vi "set led intensity.vi"(0 "WindowHandle in":T1, 2 "Abort Ref":refnum<vi>, 5 "HWND in":u32, 7 "LED":enum16{"5", "6", "10", "13", "24", "28"}(ring), 9 "PIN setpoint":i32=100, 11 "error in":errorcluster) -> (4 "WindowHandle out":T1, 6 "HWND out":u32, 15 "error out":errorcluster)   [LabVIEW 2018]
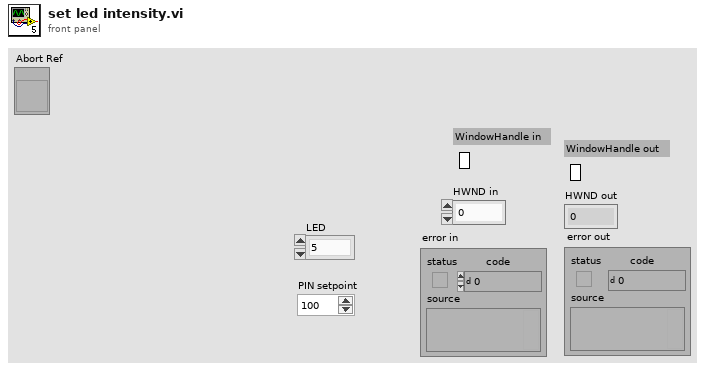
[diagram p1: front panel]
types:
  T1 = typedef "WindowHandle" = refnum<k1>
  T2 = enum16{"titlebar", "led 5", "led 6", "led 10", "led 13", "led 24", "led 28", "set PIN setpoint", "set Avg points", "set LED freq", "set LED DAC", "Toggle auto control", "Toggle Log to File", "LEF Gen ON", "LED Gen Off", "PIN setpoint", "avg points", "LED freq", "LED DAC"}
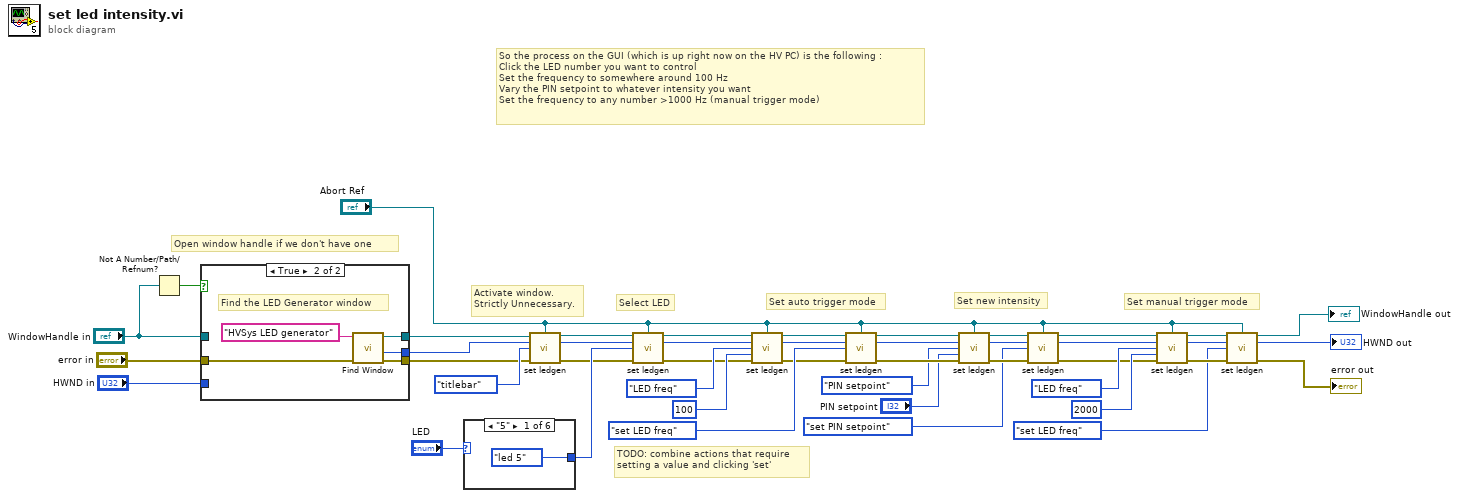
[diagram p0: block diagram]
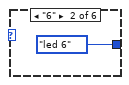
[diagram p3: hidden frame]
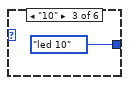
[diagram p4: hidden frame]
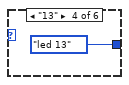
[diagram p5: hidden frame]
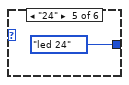
[diagram p6: hidden frame]
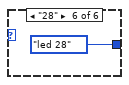
[diagram p7: hidden frame]
diagram:
  # "Open window handle if we don't have one"
  # "Set manual trigger mode"
  # "Set new intensity"
  # "Set auto trigger mode"
  # "TODO: combine actions that require\nsetting a value and clicking 'set'"
  # "Select LED"
  # "Activate window.\nStrictly Unnecessary."
  # "So the process on the GUI (which is up right now on the HV PC) is the following :\nClick the LED number you want to control\nSet the frequency to somewhere around 100 Hz\nVary the PIN setpoint to whatever intensity you want\nSet the frequency to any number >1000 Hz (manual trigger mode)"
  n1 = Not A Number/Path/Refnum?(number/path/refnum="WindowHandle in") -> (NaN/Path/Refnum?=w13:bool)
  n2 = case shown="True" w13 {
    tunnel: [w45 w51] -> w5
    tunnel: [w47 w50] -> w10
    tunnel: [w46 w49] -> w9
    tunnel: "error in" -> [w45 w48]
    tunnel: "WindowHandle in" -> [w47 _]
    tunnel: "HWND in" -> [w46 _]
    frame False {
    }
    frame True {
      # "Find the LED Generator window"
      n3 = call "Find Window.vi"("error in (no error)"=w48, "WindowName"="HVSys LED generator") -> ("error out"=w51:errorcluster, "HWND"=w49:u32, "WindowHandle"=w50:T1)  [unwired: 6 in, 1 out]
    }
  }
  n4 = case shown="\"5\"" "LED" {
    tunnel: [T2."led 5" ("Action") T2."led 6" ("Action") T2."led 10" ("Action") T2."led 13" ("Action") T2."led 24" ("Action") T2."led 28" ("Action")] -> w40
    frame "5" {
    }
    frame "6" {
    }
    frame "10" {
    }
    frame "13" {
    }
    frame "24" {
    }
    frame "28" {
    }
  }
  n5 = call "set ledgen.vi"("WindowHandle in"=w10, "Abort Ref"="Abort Ref", "HWND in"=w9, "Action"=T2."titlebar", "error in"=w5) -> ("WindowHandle out"=w43:T1, "HWND out"=w42:u32, "error out"=w4:errorcluster)  [unwired: 7 in, 1 out]
  n6 = call "set ledgen.vi"("WindowHandle in"=w43, "Abort Ref"="Abort Ref", "HWND in"=w42, "Action"=w40, "error in"=w4) -> ("WindowHandle out"=w39:T1, "HWND out"=w38:u32, "error out"=w3:errorcluster)  [unwired: 7 in, 1 out]
  n7 = call "set ledgen.vi"("WindowHandle in"=w39, "Abort Ref"="Abort Ref", "HWND in"=w38, "Action"=T2."LED freq", "New val"=100, "error in"=w3) -> ("WindowHandle out"=w35:T1, "HWND out"=w34:u32, "error out"=w2:errorcluster)  [unwired: 6 in, 1 out]
  n8 = call "set ledgen.vi"("WindowHandle in"=w35, "Abort Ref"="Abort Ref", "HWND in"=w34, "Action"=T2."set LED freq", "error in"=w2) -> ("WindowHandle out"=w32:T1, "HWND out"=w31:u32, "error out"=w30:errorcluster)  [unwired: 7 in, 1 out]
  n9 = call "set ledgen.vi"("WindowHandle in"=w32, "Abort Ref"="Abort Ref", "HWND in"=w31, "Action"=T2."PIN setpoint", "New val"="PIN setpoint", "error in"=w30) -> ("WindowHandle out"=w26:T1, "HWND out"=w25:u32, "error out"=w27:errorcluster)  [unwired: 6 in, 1 out]
  n10 = call "set ledgen.vi"("WindowHandle in"=w26, "Abort Ref"="Abort Ref", "HWND in"=w25, "Action"=T2."set PIN setpoint", "error in"=w27) -> ("WindowHandle out"=w17:T1, "HWND out"=w16:u32, "error out"=w15:errorcluster)  [unwired: 7 in, 1 out]
  n11 = call "set ledgen.vi"("WindowHandle in"=w17, "Abort Ref"="Abort Ref", "HWND in"=w16, "Action"=T2."LED freq", "New val"=2000, "error in"=w15) -> ("WindowHandle out"=w20:T1, "HWND out"=w21:u32, "error out"=w23:errorcluster)  [unwired: 6 in, 1 out]
  n12 = call "set ledgen.vi"("WindowHandle in"=w20, "Abort Ref"="Abort Ref", "HWND in"=w21, "Action"=T2."set LED freq", "error in"=w23) -> ("WindowHandle out"=→"WindowHandle out":T1, "HWND out"=→"HWND out":u32, "error out"=→"error out":errorcluster)  [unwired: 7 in, 1 out]
